vi "Avg Dist To Left Wall (SubVI).vi"   [LabVIEW 2017]
uses:
  <vilib>/Analysis/baseanly.llb/Mean (DBL).vi
  <vilib>/Analysis/NI_AALBase.lvlib
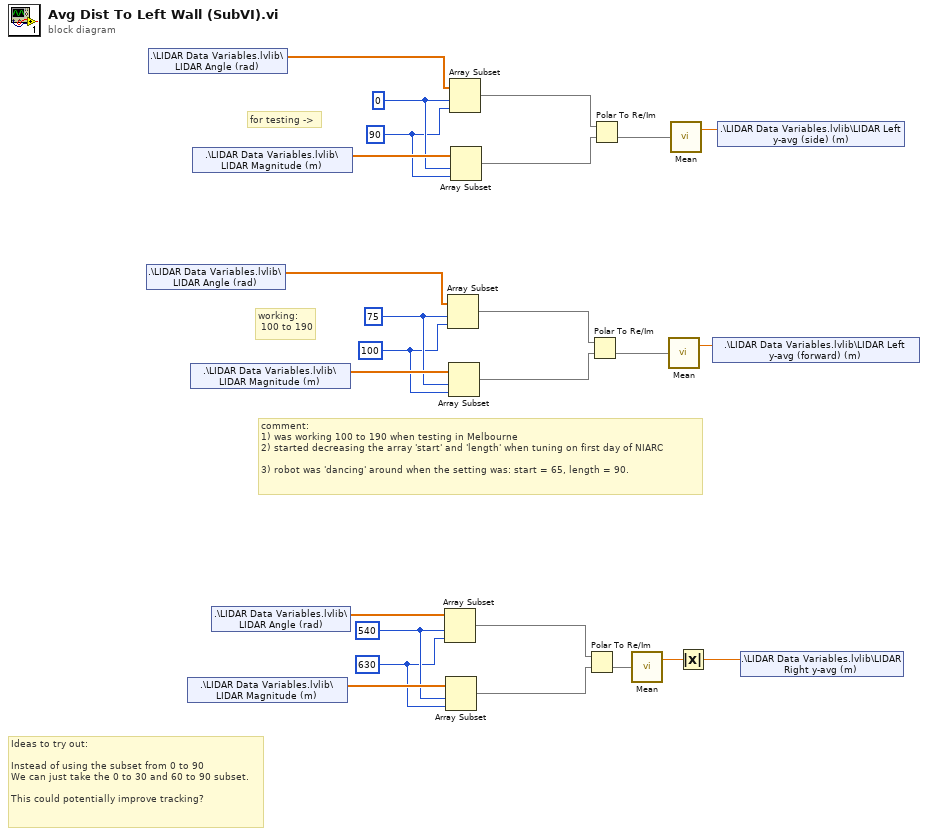
[diagram p0: block diagram]
diagram:
  w6 = 90 ("length")
  w7 = 0 ("index")
  w16 = 630 ("length")
  w17 = 540 ("index")
  w23 = 100 ("length")
  w24 = 75 ("index")
  # "comment:\n1) was working 100 to 190 when testing in Melbourne\n2) started decreasing the array 'start' and 'length' when tuning on first day of NIARC\n\n3) robot was 'dancing' around when the setting was: start = 65, length = 90."
  # "for testing ->"
  # "working:\n 100 to 190"
  # "Ideas to try out:\n\nInstead of using the subset from 0 to 90\nWe can just take the 0 to 30 and 60 to 90 subset.\n\nThis could potentially improve tracking?"
  n1 = shared-variable ".\\LIDAR Data Variables.lvlib\\LIDAR Angle (rad)"() -> (w10:dbl[])  [unwired: 1 in, 1 out]
  n2 = shared-variable ".\\LIDAR Data Variables.lvlib\\LIDAR Angle (rad)"() -> (w3:dbl[])  [unwired: 1 in, 1 out]
  n3 = shared-variable ".\\LIDAR Data Variables.lvlib\\LIDAR Magnitude (m)"() -> (w18:dbl[])  [unwired: 1 in, 1 out]
  n4 = shared-variable ".\\LIDAR Data Variables.lvlib\\LIDAR Magnitude (m)"() -> (w25:dbl[])  [unwired: 1 in, 1 out]
  n5 = shared-variable ".\\LIDAR Data Variables.lvlib\\LIDAR Magnitude (m)"() -> (w8:dbl[])  [unwired: 1 in, 1 out]
  n6 = shared-variable ".\\LIDAR Data Variables.lvlib\\LIDAR Angle (rad)"() -> (w19:dbl[])  [unwired: 1 in, 1 out]
  n7 = Array Subset(array=w19, index=w17, length=w16) -> (w15:dbl[])
  n8 = Array Subset(array=w18, index=w17, length=w16) -> (w14:dbl[])
  n9 = Array Subset(array=w10, index=w24, length=w23) -> (w22:dbl[])
  n10 = Array Subset(array=w25, index=w24, length=w23) -> (w21:dbl[])
  n11 = Array Subset(array=w3, index=w7, length=w6) -> (w5:dbl[])
  n12 = Array Subset(array=w8, index=w7, length=w6) -> (w4:dbl[])
  n13 = Polar To Re/Im(2:w14, 3:w15) -> (0:w13:dbl[])  [unwired: 1 out]
  n14 = Polar To Re/Im(2:w21, 3:w22) -> (0:w9:dbl[])  [unwired: 1 out]
  n15 = Polar To Re/Im(2:w4, 3:w5) -> (0:w2:dbl[])  [unwired: 1 out]
  n16 = call-poly <vilib>:"Mean.vi"("X"=w13) -> ("mean"=w12:dbl)  [unwired: 1 out]
  n17 = call-poly <vilib>:"Mean.vi"("X"=w9) -> ("mean"=w20:dbl)  [unwired: 1 out]
  n18 = call-poly <vilib>:"Mean.vi"("X"=w2) -> ("mean"=w1:dbl)  [unwired: 1 out]
  n19 = Absolute Value(x=w12) -> (abs(x)=w11:dbl)
  n20 = shared-variable ".\\LIDAR Data Variables.lvlib\\LIDAR Left y-avg (forward) (m)"(w20) -> ()  [unwired: 1 in, 1 out]
  n21 = shared-variable ".\\LIDAR Data Variables.lvlib\\LIDAR Left y-avg (side) (m)"(w1) -> ()  [unwired: 1 in, 1 out]
  n22 = shared-variable ".\\LIDAR Data Variables.lvlib\\LIDAR Right y-avg (m)"(w11) -> ()  [unwired: 1 in, 1 out]
